vi "Linear equation_rohit.vi"() -> ()   [LabVIEW 2009]
panel:
  out "Y":dbl
  in  "X":dbl
  in  "B":dbl
  in  "A":dbl
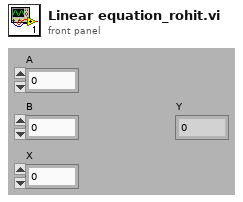
[diagram p1: front panel]
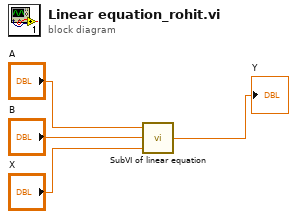
[diagram p0: block diagram]
diagram:
  n1 = call "SubVI of linear equation.vi"("X"="X", "B"="B", "A"="A") -> ("Numeric"=→"Y":dbl)
